vi "GenerateXML.vi"() -> ()   [LabVIEW 2017]
uses:
  Utils/FilePath.vi
  <vilib>/Utility/inputDevices.llb/mouseAcquire.vi
  <vilib>/xml/NI_XML.lvlib
  <resource>/objmgr/DOMUserDefRef.rc
panel:
  in  "LocalFileNames":string[](array[string])=["1A.txt", "1B.txt", "1C.txt", "1D.txt", "2A.txt", "2B.txt", "2C.txt", "2D.txt", "3A.txt", "3B.txt", "3C.txt", "3D.txt", "4A.txt", "4B.txt", "4C.txt", "4D.txt"]
  out "standard output":string
  out "standard error":string="NI Linux Real-Time (run mode)\n\nLog in with your NI-Auth credentials.\n\n"
  in  "LocalFiles":i32(listbox)=2
  in  "SaveToLocal":bool
  in  "LoadFromLocal":bool
  in  "ExportToRobot":bool
  out "XML With IDs":string="<Sequential ID=\"1\">\n</Sequential>"
  in  "Commands":i32(listbox)=-1
  out "XML":string="<Sequential>\n</Sequential>"
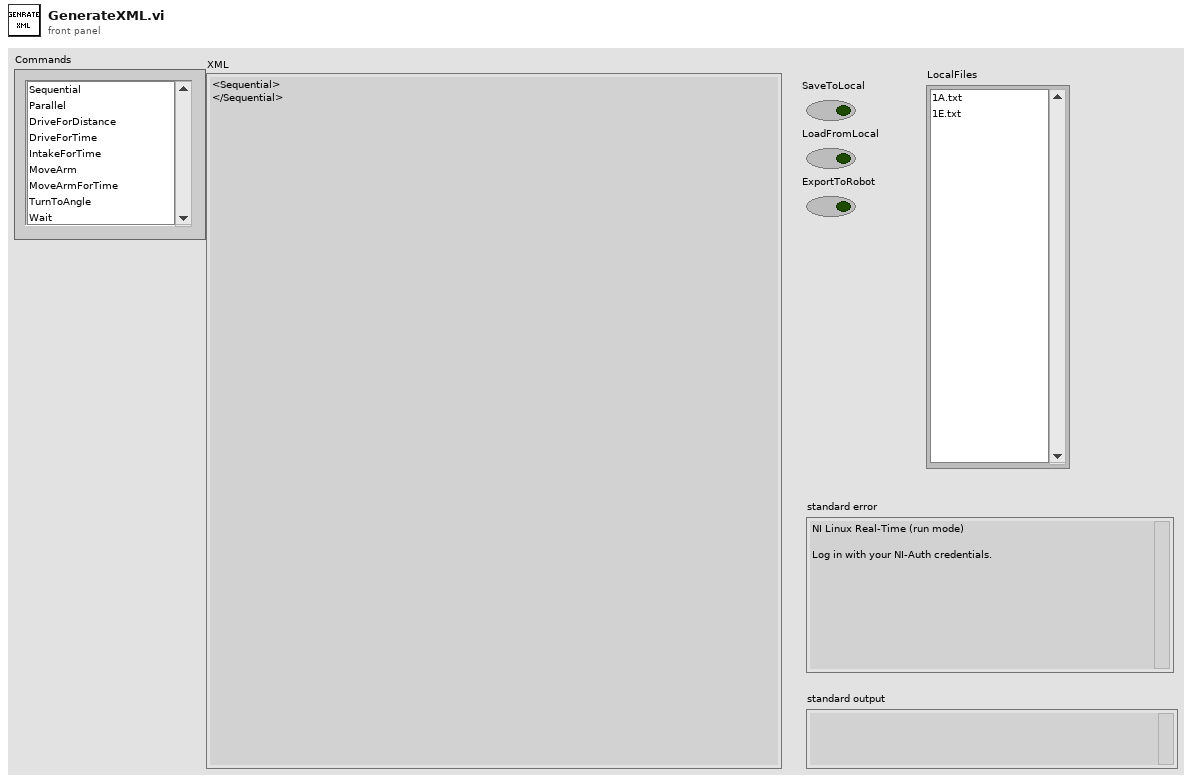
[diagram p1: front panel]
types:
  T1 = cluster{"Horizontal":i32, "Vertical":i32, "Scrolling":i32}
  T2 = typedef "eventvkey.ctl" = enum16{"ASCII", "Enter", "Return", "Shift", "Ctrl", "Alt", "Cmd", "Opt", "Caps", "NumLock", "Clear", "Break", "Up", "Down", "Left", "Right", "Insert", "Delete", "Home", "End", "PageUp", "PageDown", "Escape", "Help", "Pause", "ScrollLock", "F1", "F2", "F3", "F4", "F5", "F6", "F7", "F8", "F9", "F10", "F11", "F12", "F13", "F14", "F15", "F16", "F17", "F18", "F19", "F20", "F21", "F22", "F23", "F24", "Play", "VolumeUp", "VolumeDown", "Mute", "Two Byte Char"}
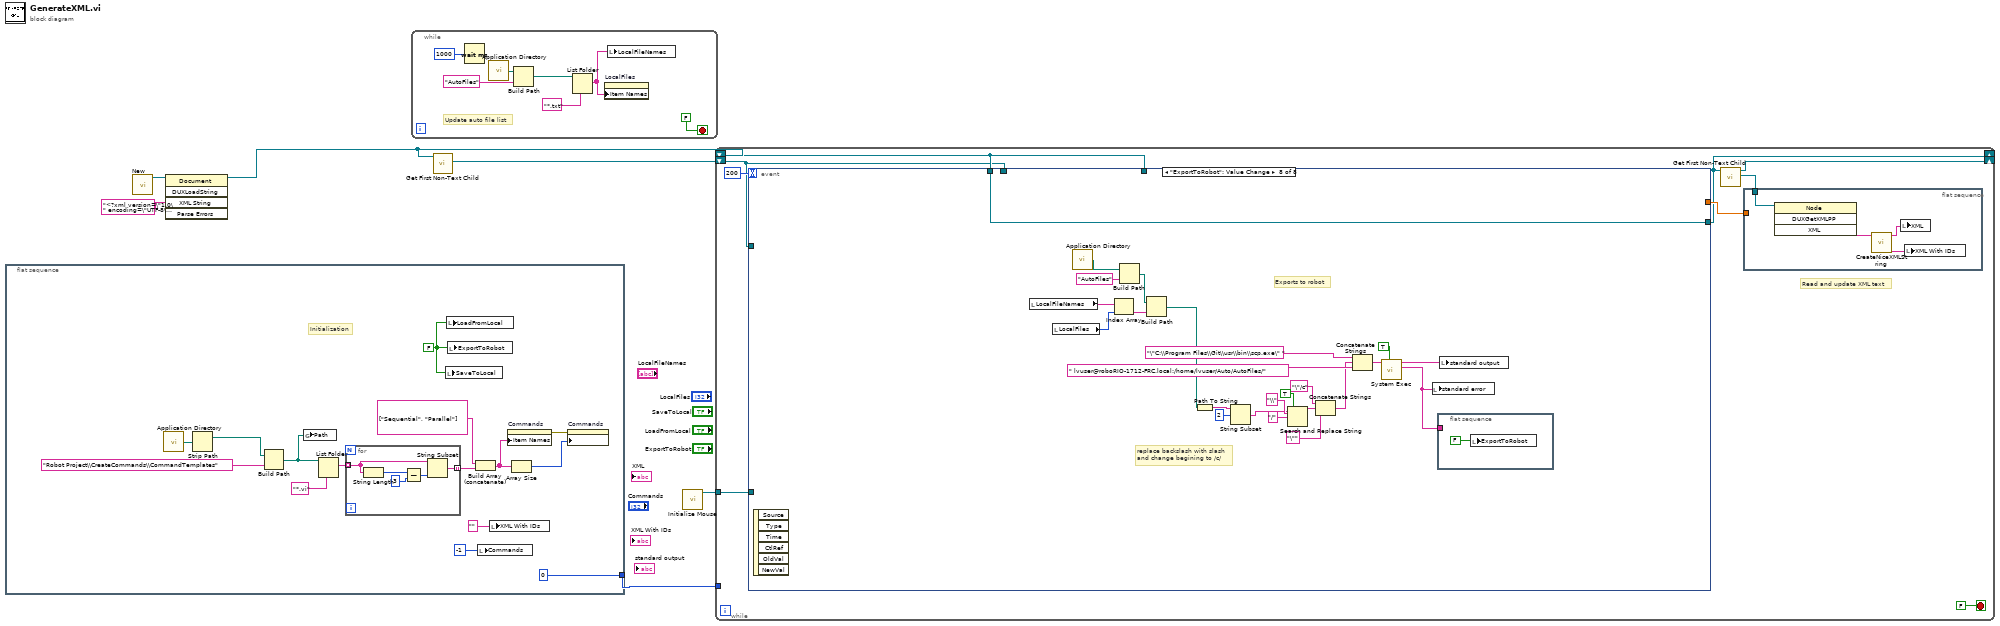
[diagram p0: block diagram]
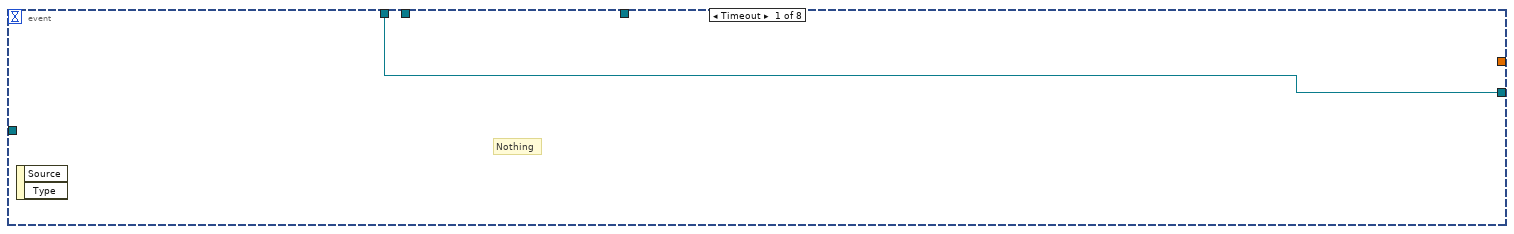
[diagram p2: hidden frame]
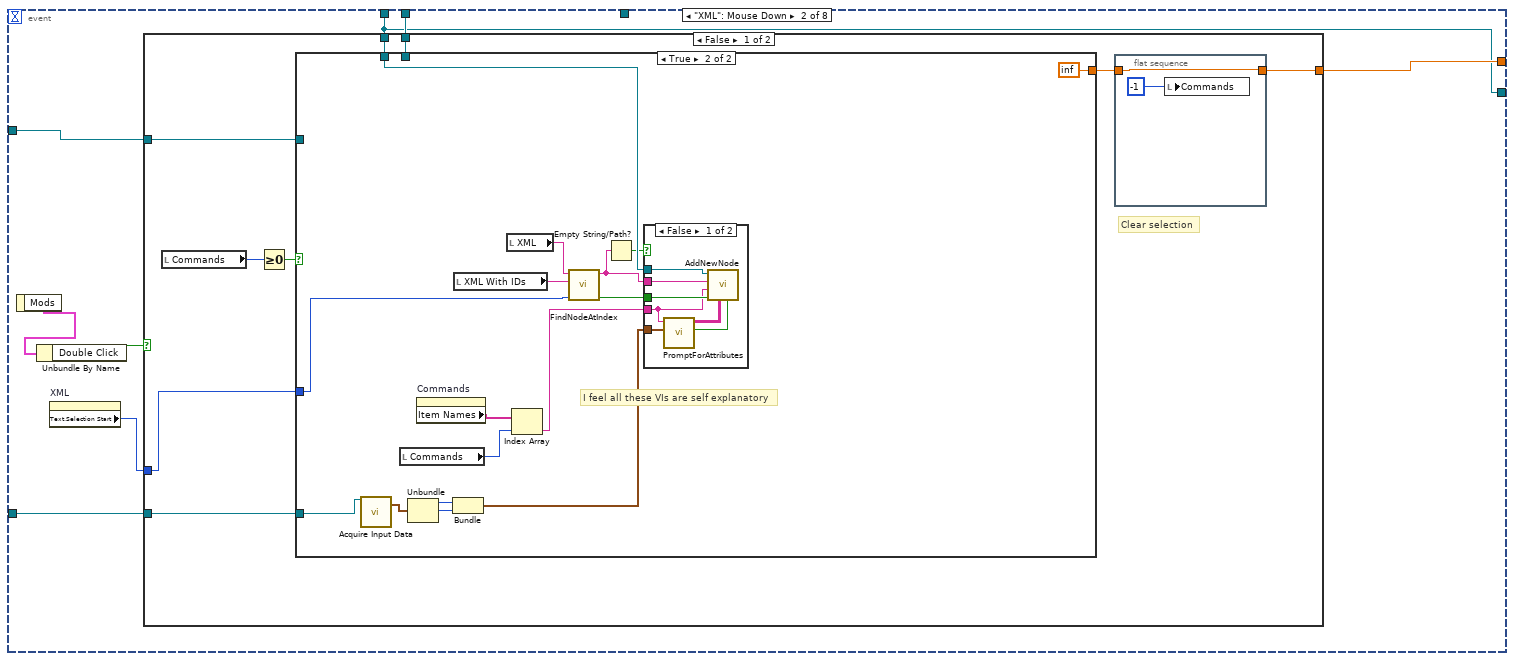
[diagram p3: hidden frame]
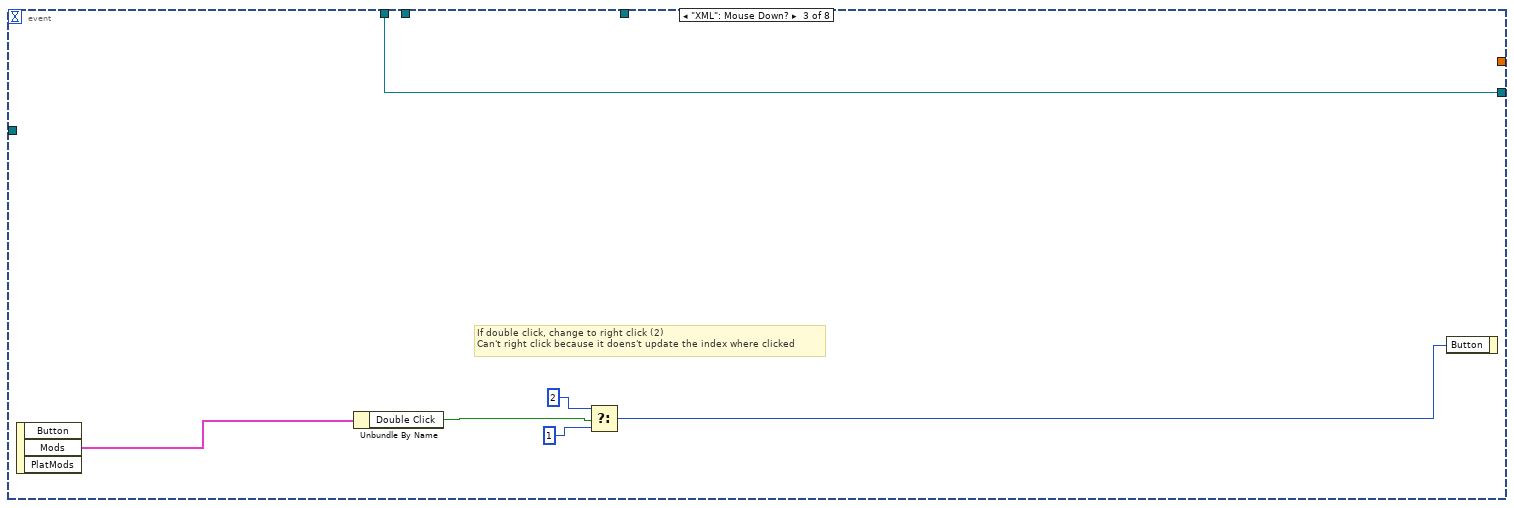
[diagram p7: hidden frame]
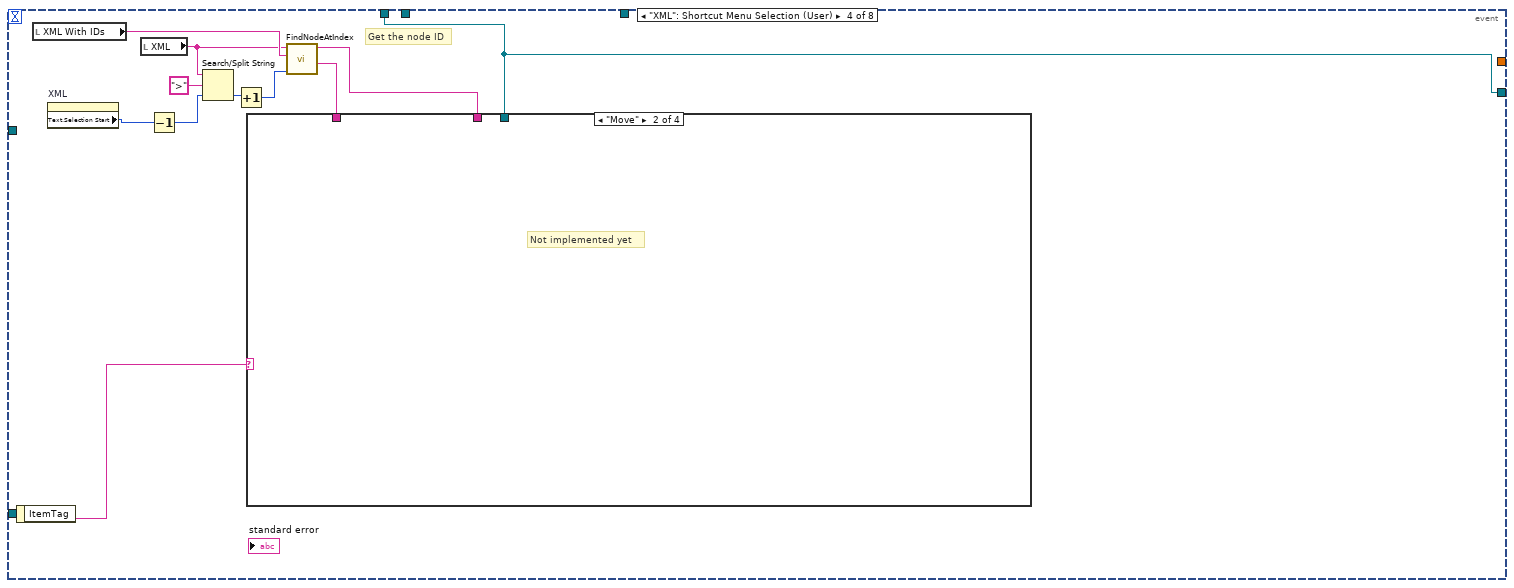
[diagram p8: hidden frame]
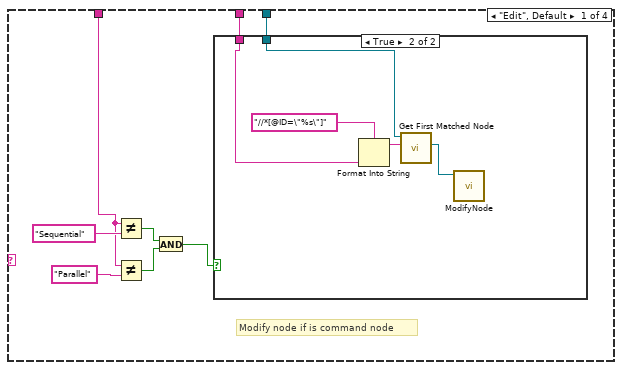
[diagram p9: hidden frame]
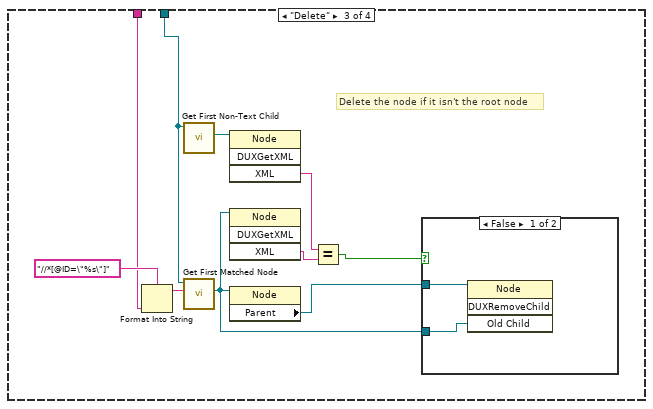
[diagram p11: hidden frame]
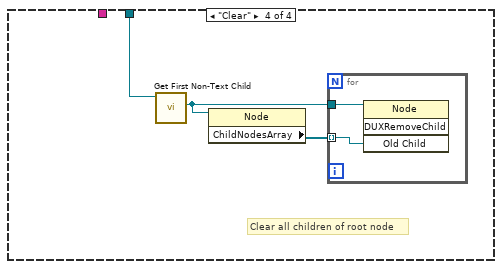
[diagram p13: hidden frame]
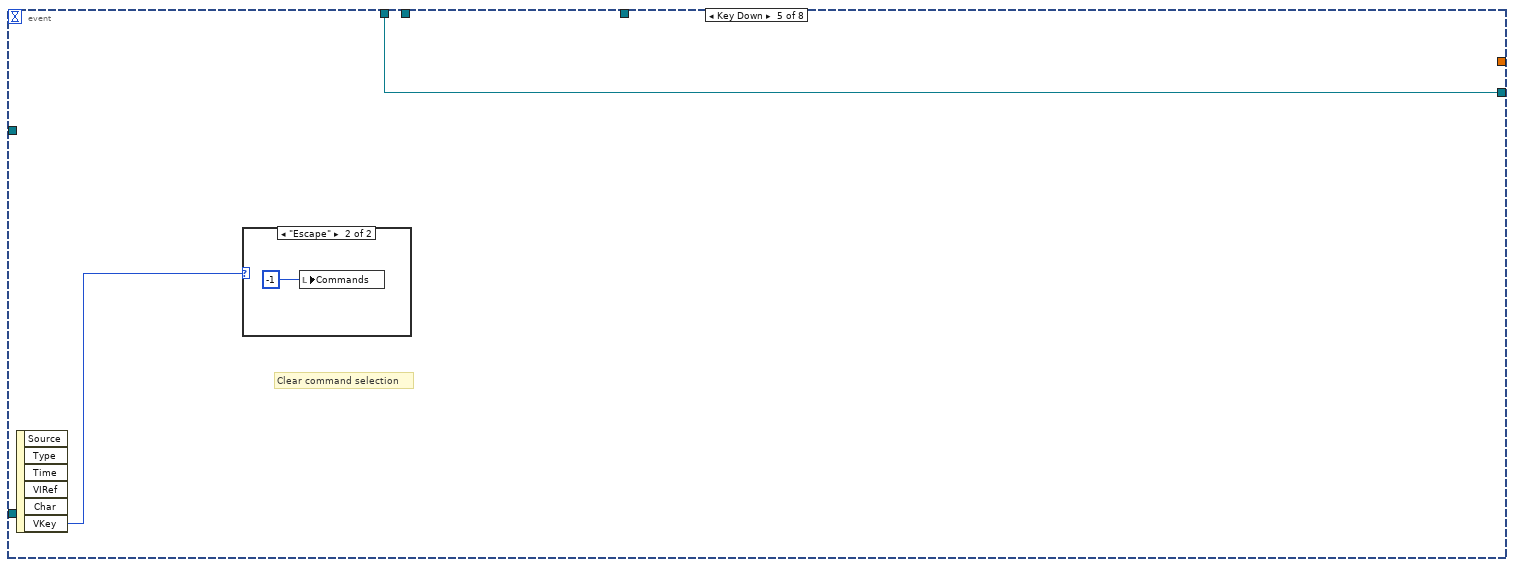
[diagram p14: hidden frame]
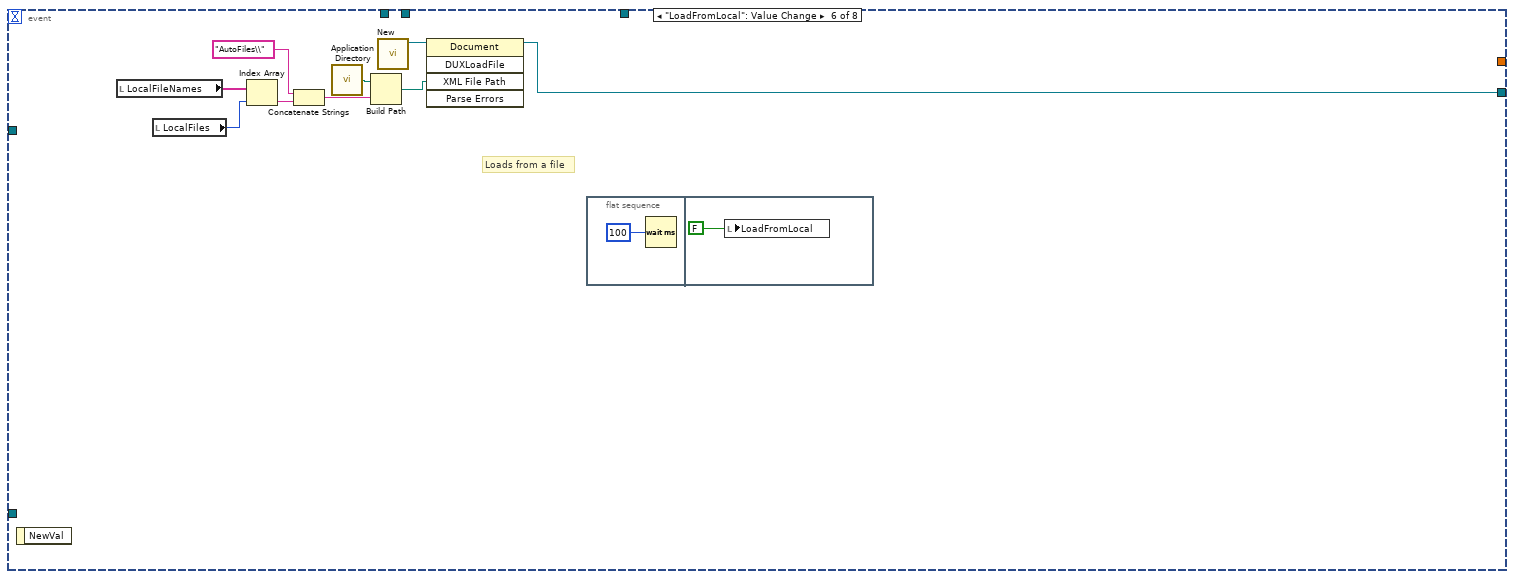
[diagram p16: hidden frame]
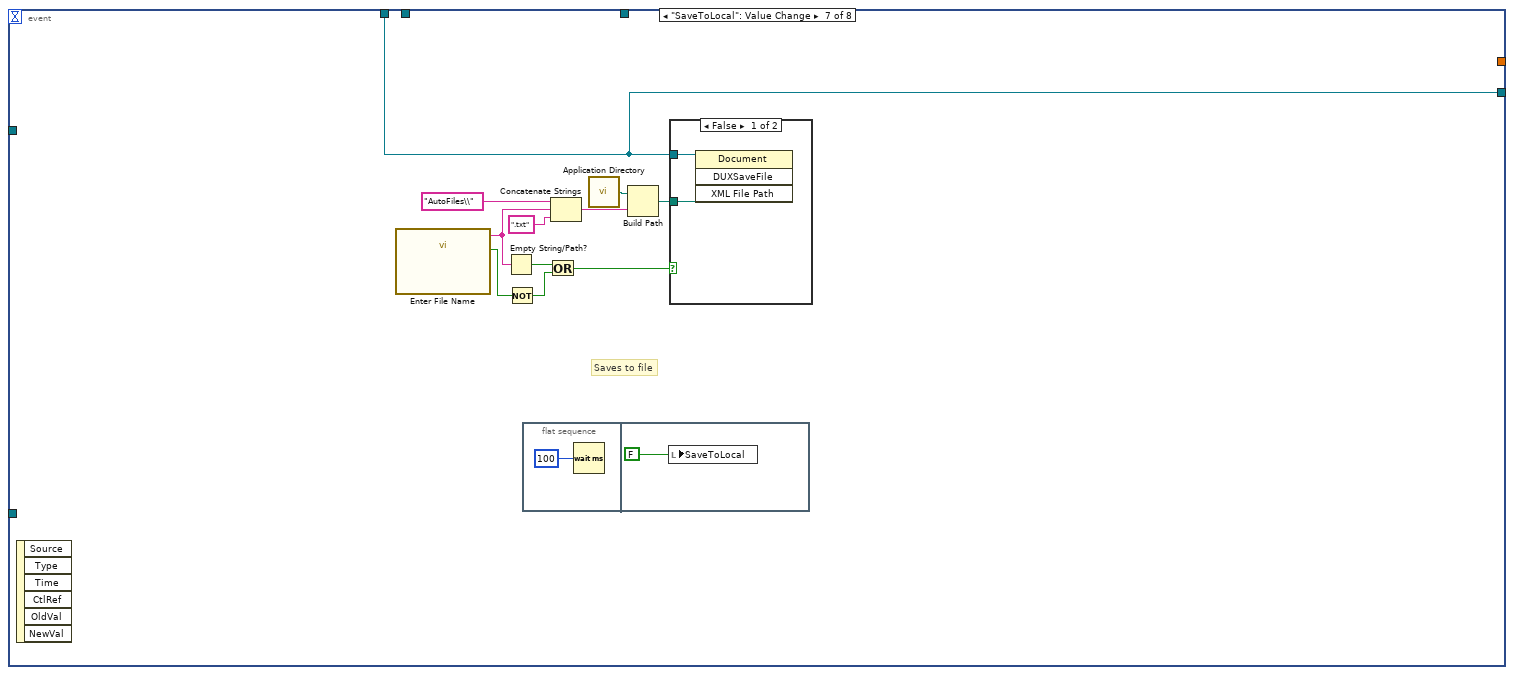
[diagram p17: hidden frame]
diagram:
  n1 = flat-sequence {
    tunnel: [0] -> w6
    frame #0 {
      w10 = FALSE ("SaveToLocal")
      # "Initialization"
      n2 = call <vilib>:"Application Directory.vi"() -> ("Application Directory"=w9:path)
      n3 = Strip Path(path=w9) -> (stripped path=w8:path)  [unwired: 1 out]
      n4 = Build Path(base path=w8, name or relative path="Robot Project\\CreateCommands\\CommandTemplates") -> (appended path=w7:path)
      n5 = global write "FilePath.vi" "Path"(w7) -> ()
      n6 = List Folder(path=w7, pattern="*.vi") -> (filenames=w14:string[])  [unwired: 2 in, 3 out]
      n7 = for {
        tunnel: w14 -> [w26] mode=indexing
        tunnel: [w22] -> w15 mode=indexing
        n8 = String Length(string=w26) -> (length=w25:i32)
        n9 = Subtract(x=w25, y=3) -> (x-y=w23:i32)
        n10 = String Subset(string=w26, length (rest)=w23) -> (substring=w22:string)  [unwired: 1 in]
      }
      n11 = local write "SaveToLocal"(w10) -> ()
      n12 = local write "LoadFromLocal"(w10) -> ()
      n13 = local write "ExportToRobot"(w10) -> ()
      n14 = Build Array (concatenate)(string[] ["Sequential", "Parallel"], w15) -> (w16:string[])
      n15 = local write "Commands"(-1 ("Active Row:Active Row Number")) -> ()
      n16 = local write "XML With IDs"("" ("XML With IDs")) -> ()
      n17 = property on="Commands" class="LstBox (strict)"("Item Names"=w16) -> (error out=w18:errorcluster)  [unwired: 2 in, 1 out]
      n18 = Array Size(array=w16) -> (size(s)=w17:i32)
      n19 = property on="Commands" class="LstBox (strict)"(error in=w18, "Number of Rows"=w17) -> ()  [unwired: 1 in, 2 out]
    }
  }
  n20 = call <vilib>:"New.vi"() -> ("DOM document out"=w5:refnum<k20>)  [unwired: 8 in, 1 out]
  n21 = invoke class="Document" method="DUXLoadString"(reference=w5, "XML String"="<?xml version=\"1.0\" encoding=\"UTF-8\"?><Sequential ID=\"1\"></Sequential>") -> (reference out=w4:refnum<k20>)  [unwired: 3 in, 4 out]
  n22 = while {
    stop <- FALSE stop-if-true
    # "Update auto file list"
    n23 = Wait (ms)(milliseconds to wait=u32 1000) -> ()  [unwired: 1 out]
    n24 = call <vilib>:"Application Directory.vi"() -> ("Application Directory"=w28:path)
    n25 = Build Path(base path=w28, name or relative path="AutoFiles") -> (appended path=w33:path)
    n26 = List Folder(path=w33, pattern="*.txt") -> (filenames=w27:string[])  [unwired: 2 in, 3 out]
    n27 = property on="LocalFiles" class="LstBox (strict)"("Item Names"=w27) -> ()  [unwired: 2 in, 2 out]
    n28 = local write "LocalFileNames"(w27) -> ()
  }
  n29 = call <vilib>:"Get First Non-Text Child.vi"("node in"=w4) -> ("child node"=w3:refnum<k20>)  [unwired: 7 in, 3 out]
  n30 = call <vilib>:"Initialize Mouse.vi"() -> ("device ID"=w2:refnum<k1>)  [unwired: 10 in, 1 out]
  n31 = while {
    tunnel: w6 -> [_]
    shift-right: [w34] -> _
    shift-left: w4 -> [w38]
    shift-right: [w36] -> _
    shift-left: w3 -> [w37]
    tunnel: w2 -> [w39]
    stop <- FALSE stop-if-true
    # "Read and update XML text"
    n32 = event shown="[7] \"ExportToRobot\": Value Change" {
      selector: _ -> [_ _ _ _ _ _ _ _]
      dyn-events: _ -> [_ _ _ _ _ _ _ _]
      timeout: 200 -> [_ _ _ _ _ _ _ _]
      tunnel: w37 -> [_ w55 _ _ _ _ _ _]
      tunnel: w38 -> [w47 w48 w90 w96 w137 _ w151 w167]
      tunnel: w37 -> [_ w54 _ _ _ _ _ _]
      tunnel: [_ w53 _ _ _ _ _ _] -> w40
      tunnel: w39 -> [_ w52 _ _ _ _ _ _]
      tunnel: w38 -> [_ _ _ _ _ _ _ _]
      tunnel: [w47 w48 w90 w96 w137 w140 w151 w167] -> w34
      event Timeout {
        # "Nothing"
        n33 = event-data() -> ()  [unwired: 1 in, 2 out]
      }
      event "XML": Mouse Down {
        n34 = event-data() -> ("Mods"=w51:cluster{"Double Click":bool, "Menu Key":bool})  [unwired: 1 in]
        n35 = Unbundle By Name(w51) -> ("Double Click"=w50:bool)
        n36 = property on="XML" class="Str"() -> ("Text.Selection Start"=w49:u32)  [unwired: 2 in, 2 out]
        n37 = case shown="False" w50 {
          tunnel: w55 -> [w62 _]
          tunnel: w48 -> [w61 _]
          tunnel: w54 -> [w60 _]
          tunnel: [w58 _] -> w53
          tunnel: w52 -> [w57 _]
          tunnel: w49 -> [w56 _]
          frame False {
            # "Clear selection"
            n38 = local read "Commands"() -> (w64:i32)
            n39 = Greater Or Equal To 0?(x=w64) -> (x >= 0?=w63:bool)
            n40 = case shown="True" w63 {
              tunnel: w62 -> [_ _]
              tunnel: w61 -> [_ w73]
              tunnel: w60 -> [_ _]
              tunnel: w56 -> [_ w77]
              tunnel: [_ inf] -> w59
              tunnel: w57 -> [_ w71]
              frame False {
              }
              frame True {
                # "I feel all these VIs are self explanatory"
                n41 = call-poly <vilib>:"Acquire Input Data.vi"("device ID"=w71) -> ("axis info"=w70:T1)  [unwired: 15 in, 3 out]
                n42 = local read "Commands"() -> (w79:i32)
                n43 = Unbundle(w70) -> ("Horizontal"=w69:i32, "Vertical"=w68:i32)  [unwired: 1 out]
                n44 = property on="Commands" class="LstBox (strict)"() -> ("Item Names"=w80:string[])  [unwired: 2 in, 2 out]
                n45 = Bundle("Horizontal"=w69, "Vertical"=w68) -> (w65:cluster{"Horizontal":i32, "Vertical":i32})  [unwired: 1 in]
                n46 = local read "XML With IDs"() -> (w76:string)
                n47 = local read "XML"() -> (w75:string)
                n48 = Index Array(array=w80, index=w79) -> (element=w72:string)
                n49 = call "FindNodeAtIndex.vi"("ClickIndex"=w77, "XML with IDs"=w76, "XML In"=w75) -> ("Insert as child not sibling"=w74:bool, "Node ID"=w67:string)  [unwired: 6 in, 1 out]
                n50 = Empty String/Path?(string/path=w67) -> (empty?=w66:bool)
                n51 = case shown="False" w66 {
                  tunnel: w74 -> [w87 _]
                  tunnel: w73 -> [w86 _]
                  tunnel: w72 -> [w83 _]
                  tunnel: w67 -> [w85 _]
                  tunnel: w65 -> [w84 _]
                  frame False {
                    n52 = call "PromptForAttributes.vi"("Mouse Coords"=w84, "New Node Name"=w83) -> ("Canceled"=w82:bool, "Attributes"=w81:string[][])  [unwired: 8 in]
                    n53 = call "AddNewNode.vi"("Cancel"=w82, "Attributes"=w81, "Insert As Child"=w87, "New Node Name"=w83, "Node ID"=w85, "DOM document"=w86) -> ()  [unwired: 6 in]
                  }
                  frame True {
                  }
                }
              }
            }
            n54 = flat-sequence {
              tunnel: w59 -> [w88]
              tunnel: [w88] -> w58
              frame #0 {
                n55 = local write "Commands"(-1 ("Active Row:Active Row Number")) -> ()
              }
            }
          }
          frame True {
            # "Leave double clicking to that other event case"
          }
        }
      }
      event "XML": Mouse Down? {
        # "If double click, change to right click (2)\nCan't right click because it doens't update the index where clicked"
        n56 = event-data() -> ("Mods"=w95:cluster{"Double Click":bool, "Menu Key":bool})  [unwired: 1 in, 2 out]
        n57 = Unbundle By Name(w95) -> ("Double Click"=w94:bool)
        n58 = Select(t=u16 2 ("Button"), s=w94, f=u16 1 ("Button")) -> (s? t:f=w91:u16)
        n59 = event-data("Button"=w91) -> ()  [unwired: 1 in, 1 out]
      }
      event "XML": Shortcut Menu Selection (User) {
        # "Get the node ID"
        n60 = event-data() -> ("ItemTag"=w101:string)  [unwired: 1 in]
        n61 = local read "XML With IDs"() -> (w98:string)
        n62 = property on="XML" class="Str"() -> ("Text.Selection Start"=w106:u32)  [unwired: 2 in, 2 out]
        n63 = local read "XML"() -> (w97:string)
        n64 = Decrement(x=w106) -> (x-1=w104:u32)
        n65 = Search/Split String(string=w97, search string/char (-)=">", offset (0)=w104) -> (offset of match=w102:i32)  [unwired: 2 out]
        n66 = Increment(x=w102) -> (x+1=w103:i32)
        n67 = call "FindNodeAtIndex.vi"("ClickIndex"=w103, "XML with IDs"=w98, "XML In"=w97) -> ("Node Name"=w99:string, "Node ID"=w100:string)  [unwired: 6 in, 1 out]
        n68 = case shown="\"Move\"" w101 {
          tunnel: w100 -> [w114 _ w127 _]
          tunnel: w96 -> [w113 _ w120 w134]
          tunnel: w99 -> [w110 _ _ _]
          frame "Edit", Default {
            # "Modify node if is command node"
            n69 = Not Equal?(x=w110, y="Sequential") -> (x != y?=w111:bool)
            n70 = Not Equal?(x=w110, y="Parallel") -> (x != y?=w108:bool)
            n71 = And(x=w111, y=w108) -> (x .and. y?=w107:bool)
            n72 = case shown="True" w107 {
              tunnel: w114 -> [_ w117]
              tunnel: w113 -> [_ w115]
              frame False {
              }
              frame True {
                n73 = Format Into String(format string="//*[@ID=\"%s\"]", w117) -> (resulting string=w119:string)  [unwired: 2 in, 1 out]
                n74 = call <vilib>:"Get First Matched Node.vi"("XPath expression"=w119, "node in"=w115) -> ("node result"=w116:refnum<k20>)  [unwired: 7 in, 2 out]
                n75 = call "ModifyNode.vi"("Node"=w116) -> ()  [unwired: 11 in]
              }
            }
          }
          frame "Move" {
            # "Not implemented yet"
          }
          frame "Delete" {
            # "Delete the node if it isn't the root node"
            n76 = Format Into String(format string="//*[@ID=\"%s\"]", w127) -> (resulting string=w129:string)  [unwired: 2 in, 1 out]
            n77 = call <vilib>:"Get First Non-Text Child.vi"("node in"=w120) -> ("child node"=w125:refnum<k20>)  [unwired: 7 in, 3 out]
            n78 = call <vilib>:"Get First Matched Node.vi"("XPath expression"=w129, "node in"=w120) -> ("node result"=w123:refnum<k20>)  [unwired: 7 in, 2 out]
            n79 = invoke class="Node" method="DUXGetXML"(reference=w125) -> ("XML"=w124:string)  [unwired: 3 in, 3 out]
            n80 = invoke class="Node" method="DUXGetXML"(reference=w123) -> ("XML"=w122:string)  [unwired: 3 in, 3 out]
            n81 = property class="Node"(reference=w123) -> ("Parent"=w126:refnum<k20>)  [unwired: 1 in, 2 out]
            n82 = Equal?(x=w124, y=w122) -> (x = y?=w121:bool)
            n83 = case shown="False" w121 {
              tunnel: w126 -> [w131 _]
              tunnel: w123 -> [w130 _]
              frame False {
                n84 = invoke class="Node" method="DUXRemoveChild"(reference=w131, "Old Child"=w130) -> ()  [unwired: 2 in, 4 out]
              }
              frame True {
              }
            }
          }
          frame "Clear" {
            # "Clear all children of root node"
            n85 = call <vilib>:"Get First Non-Text Child.vi"("node in"=w134) -> ("child node"=w132:refnum<k20>)  [unwired: 7 in, 3 out]
            n86 = property class="Node"(reference=w132) -> ("ChildNodesArray"=w133:refnum<k20>[])  [unwired: 1 in, 2 out]
            n87 = for {
              tunnel: w132 -> [w136]
              tunnel: w133 -> [w135] mode=indexing
              n88 = invoke class="Node" method="DUXRemoveChild"(reference=w136, "Old Child"=w135) -> ()  [unwired: 2 in, 4 out]
            }
          }
        }
      }
      event Key Down {
        # "Clear command selection"
        n89 = event-data() -> ("VKey"=w138:T2)  [unwired: 1 in, 5 out]
        n90 = case shown="\"Escape\"" w138 {
          frame "ASCII", Default {
          }
          frame "Escape" {
            n91 = local write "Commands"(-1 ("Active Row:Active Row Number")) -> ()
          }
        }
      }
      event "LoadFromLocal": Value Change {
        # "Loads from a file"
        n92 = event-data() -> ()  [unwired: 1 in, 1 out]
        n93 = local read "LocalFileNames"() -> (w148:string[])
        n94 = local read "LocalFiles"() -> (w147:i32)
        n95 = Index Array(array=w148, index=w147) -> (element=w143:string)
        n96 = Concatenate Strings("AutoFiles\\" ("string"), w143) -> (w141:string)
        n97 = call <vilib>:"Application Directory.vi"() -> ("Application Directory"=w146:path)
        n98 = Build Path(base path=w146, name or relative path=w141) -> (appended path=w145:path)
        n99 = call <vilib>:"New.vi"() -> ("DOM document out"=w144:refnum<k20>)  [unwired: 8 in, 1 out]
        n100 = invoke class="Document" method="DUXLoadFile"(reference=w144, "XML File Path"=w145) -> (reference out=w140:refnum<k20>)  [unwired: 3 in, 4 out]
        n101 = flat-sequence {
          frame #0 {
            n102 = Wait (ms)(milliseconds to wait=u32 100) -> ()  [unwired: 1 out]
          }
          frame #1 {
            n103 = local write "LoadFromLocal"(FALSE ("SaveToLocal")) -> ()
          }
        }
      }
      event "SaveToLocal": Value Change {
        # "Saves to file"
        n104 = event-data() -> ()  [unwired: 1 in, 6 out]
        n105 = call "Enter File Name"() -> ("File Name"=w153:string, "Enter"=w159:bool)  [unwired: 17 in, 1 out]
        n106 = Empty String/Path?(string/path=w153) -> (empty?=w161:bool)
        n107 = Not(x=w159) -> (.not. x?=w160:bool)
        n108 = flat-sequence {
          frame #0 {
            n109 = Wait (ms)(milliseconds to wait=u32 100) -> ()  [unwired: 1 out]
          }
          frame #1 {
            n110 = local write "SaveToLocal"(FALSE ("SaveToLocal")) -> ()
          }
        }
        n111 = Or(x=w161, y=w160) -> (x .or. y?=w152:bool)
        n112 = Concatenate Strings("AutoFiles\\" ("name or relative path"), w153, ".txt" ("string")) -> (w156:string)
        n113 = call <vilib>:"Application Directory.vi"() -> ("Application Directory"=w155:path)
        n114 = Build Path(base path=w155, name or relative path=w156) -> (appended path=w154:path)
        n115 = case shown="False" w152 {
          tunnel: w151 -> [w163 _]
          tunnel: w154 -> [w162 _]
          frame False {
            n116 = invoke class="Document" method="DUXSaveFile"(reference=w163, "XML File Path"=w162) -> ()  [unwired: 2 in, 4 out]
          }
          frame True {
          }
        }
      }
      event "ExportToRobot": Value Change {
        # "Exports to robot"
        # "replace backslash with slash\nand change begining to /c/"
        n117 = event-data() -> ()  [unwired: 1 in, 6 out]
        n118 = local read "LocalFileNames"() -> (w187:string[])
        n119 = local read "LocalFiles"() -> (w186:i32)
        n120 = call <vilib>:"Application Directory.vi"() -> ("Application Directory"=w166:path)
        n121 = Index Array(array=w187, index=w186) -> (element=w188:string)
        n122 = Build Path(base path=w166, name or relative path="AutoFiles") -> (appended path=w189:path)
        n123 = Build Path(base path=w189, name or relative path=w188) -> (appended path=w170:path)
        n124 = Path To String(path=w170) -> (string=w177:string)
        n125 = String Subset(string=w177, offset (0)=2) -> (substring=w175:string)  [unwired: 1 in]
        n126 = Search and Replace String(replace all?=TRUE ("replace all? (F)"), input string=w175, search string="\\", replace string="/" ("replace string (\"\")")) -> (result string=w174:string)  [unwired: 4 in, 3 out]
        n127 = Concatenate Strings("\"/c" ("string"), w174, "\"" ("string")) -> (w172:string)
        n128 = Concatenate Strings("\"C:\\Program Files\\Git\\usr\\bin\\scp.exe\" " ("command line"), w172, " lvuser@roboRIO-1712-FRC.local:/home/lvuser/Auto/AutoFiles/" ("string")) -> (w181:string)
        n129 = call <vilib>:"System Exec.vi"("wait until completion? (T)"=TRUE, "command line"=w181) -> ("standard error"=w168:string, "standard output"=w169:string)  [unwired: 6 in, 2 out]
        n130 = local write "standard error"(w168) -> ()
        n131 = flat-sequence {
          tunnel: w168 -> [_]
          frame #0 {
            n132 = local write "ExportToRobot"(FALSE ("ExportToRobot")) -> ()
          }
        }
        n133 = local write "standard output"(w169) -> ()
      }
    }
    n134 = call <vilib>:"Get First Non-Text Child.vi"("node in"=w34) -> ("child node"=w35:refnum<k20>, "node out"=w36:refnum<k20>)  [unwired: 7 in, 2 out]
    n135 = flat-sequence {
      tunnel: w40 -> [_]
      tunnel: w35 -> [w43]
      frame #0 {
        n136 = invoke class="Node" method="DUXGetXMLPP"(reference=w43) -> ("XML"=w44:string)  [unwired: 3 in, 3 out]
        n137 = call "CreateNiceXMLString.vi"("XML In"=w44) -> ("XML String With IDs"=w45:string, "XML String Human Readable"=w46:string)  [unwired: 9 in]
        n138 = local write "XML"(w46) -> ()
        n139 = local write "XML With IDs"(w45) -> ()
      }
    }
  }
